vi "LWXPS_PositionerDriverFiltersGet.vi"(0 "XPS Reference IN":refnum<k24>, 7 "Positioner Name":string, 11 "LabVIEW error IN":errorcluster) -> (2 "XPS Reference OUT":refnum<k24>, 3 "Returned error code":i32, 4 "Driver KI":dbl, 6 "Driver notch frequency":dbl, 8 "Driver notch bandwidth":dbl, 10 "Driver notch gain":dbl, 13 "LabVIEW error OUT":errorcluster, 14 "XPS Error String":string, 15 "Driver lowpass frequency":dbl)   [LabVIEW 2014]
uses:
  D:/XPSQ8_LabView_Library/Development/Source/Dll/Newport.XPS.CommandInterface.dll
  Dll/Newport.XPS.CommandInterface.dll
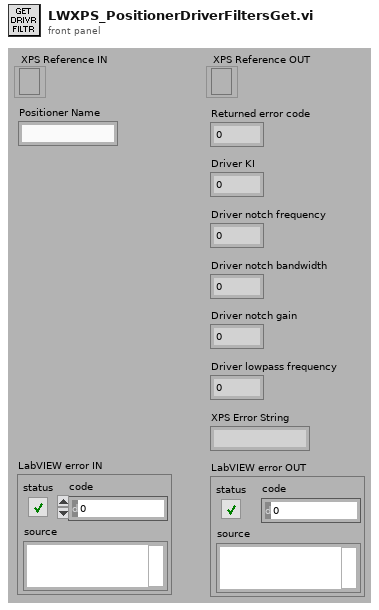
[diagram p1: front panel]
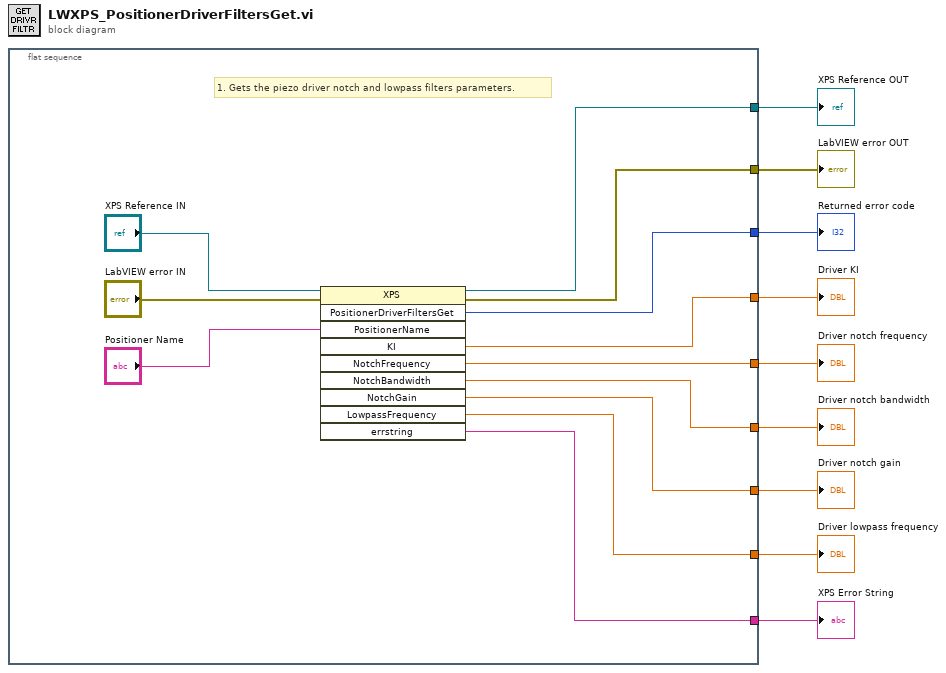
[diagram p0: block diagram]
diagram:
  n1 = flat-sequence {
    tunnel: [w15] -> w1
    tunnel: [w20] -> w9
    tunnel: [w19] -> w8
    tunnel: [w18] -> w7
    tunnel: [w14] -> w5
    tunnel: [w13] -> w4
    tunnel: [w12] -> w3
    tunnel: [w11] -> w2
    tunnel: [w10] -> w6
    frame #0 {
      # "1. Gets the piezo driver notch and lowpass filters parameters."
      n2 = invoke class="XPS" method="PositionerDriverFiltersGet"(reference="XPS Reference IN", error in="LabVIEW error IN", "PositionerName"="Positioner Name") -> (reference out=w20:refnum<k24>, error out=w19:errorcluster, "PositionerDriverFiltersGet"=w18:i32, "KI"=w15:dbl, "NotchFrequency"=w14:dbl, "NotchBandwidth"=w13:dbl, "NotchGain"=w12:dbl, "LowpassFrequency"=w11:dbl, "errstring"=w10:string)  [unwired: 7 in, 1 out]
    }
  }
  "XPS Error String" <- w6
  "XPS Reference OUT" <- w9
  "LabVIEW error OUT" <- w8
  "Returned error code" <- w7
  "Driver notch frequency" <- w5
  "Driver notch bandwidth" <- w4
  "Driver notch gain" <- w3
  "Driver lowpass frequency" <- w2
  "Driver KI" <- w1
